vi "Save Data (SubVI).vi"(0 "Save Enable":bool, 5 "Save Interval [sec]":dbl=1.0 min=0.0 step=0.1, 7 "File Name":string, 9 "Folder Location":path, 11 "Data Array (Row)":string[](array[string]), 12 "Column Header Array":string[](array[string]), 13 "Title Block":string[][](array[string]), 14 "External Save Signal":bool) -> (4 "File Path":path, 8 "Row Count":u16, 15 "Save Error":errorcluster)   [LabVIEW 2012]
panel:
  # "SAVE DATA\nCreated by Blake Otting \nLast Update 7-11-2013"
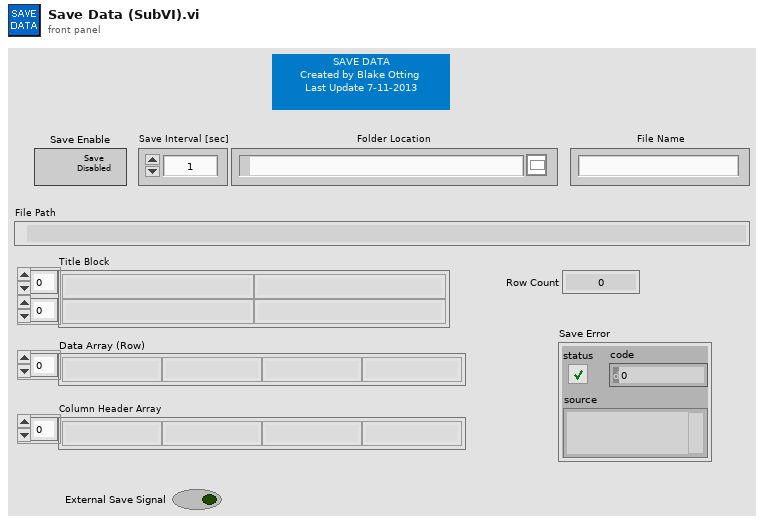
[diagram p1: front panel]
types:
  T1 = enum16{"open", "replace", "create", "open or create", "replace or create", "replace or create with confirmation"}
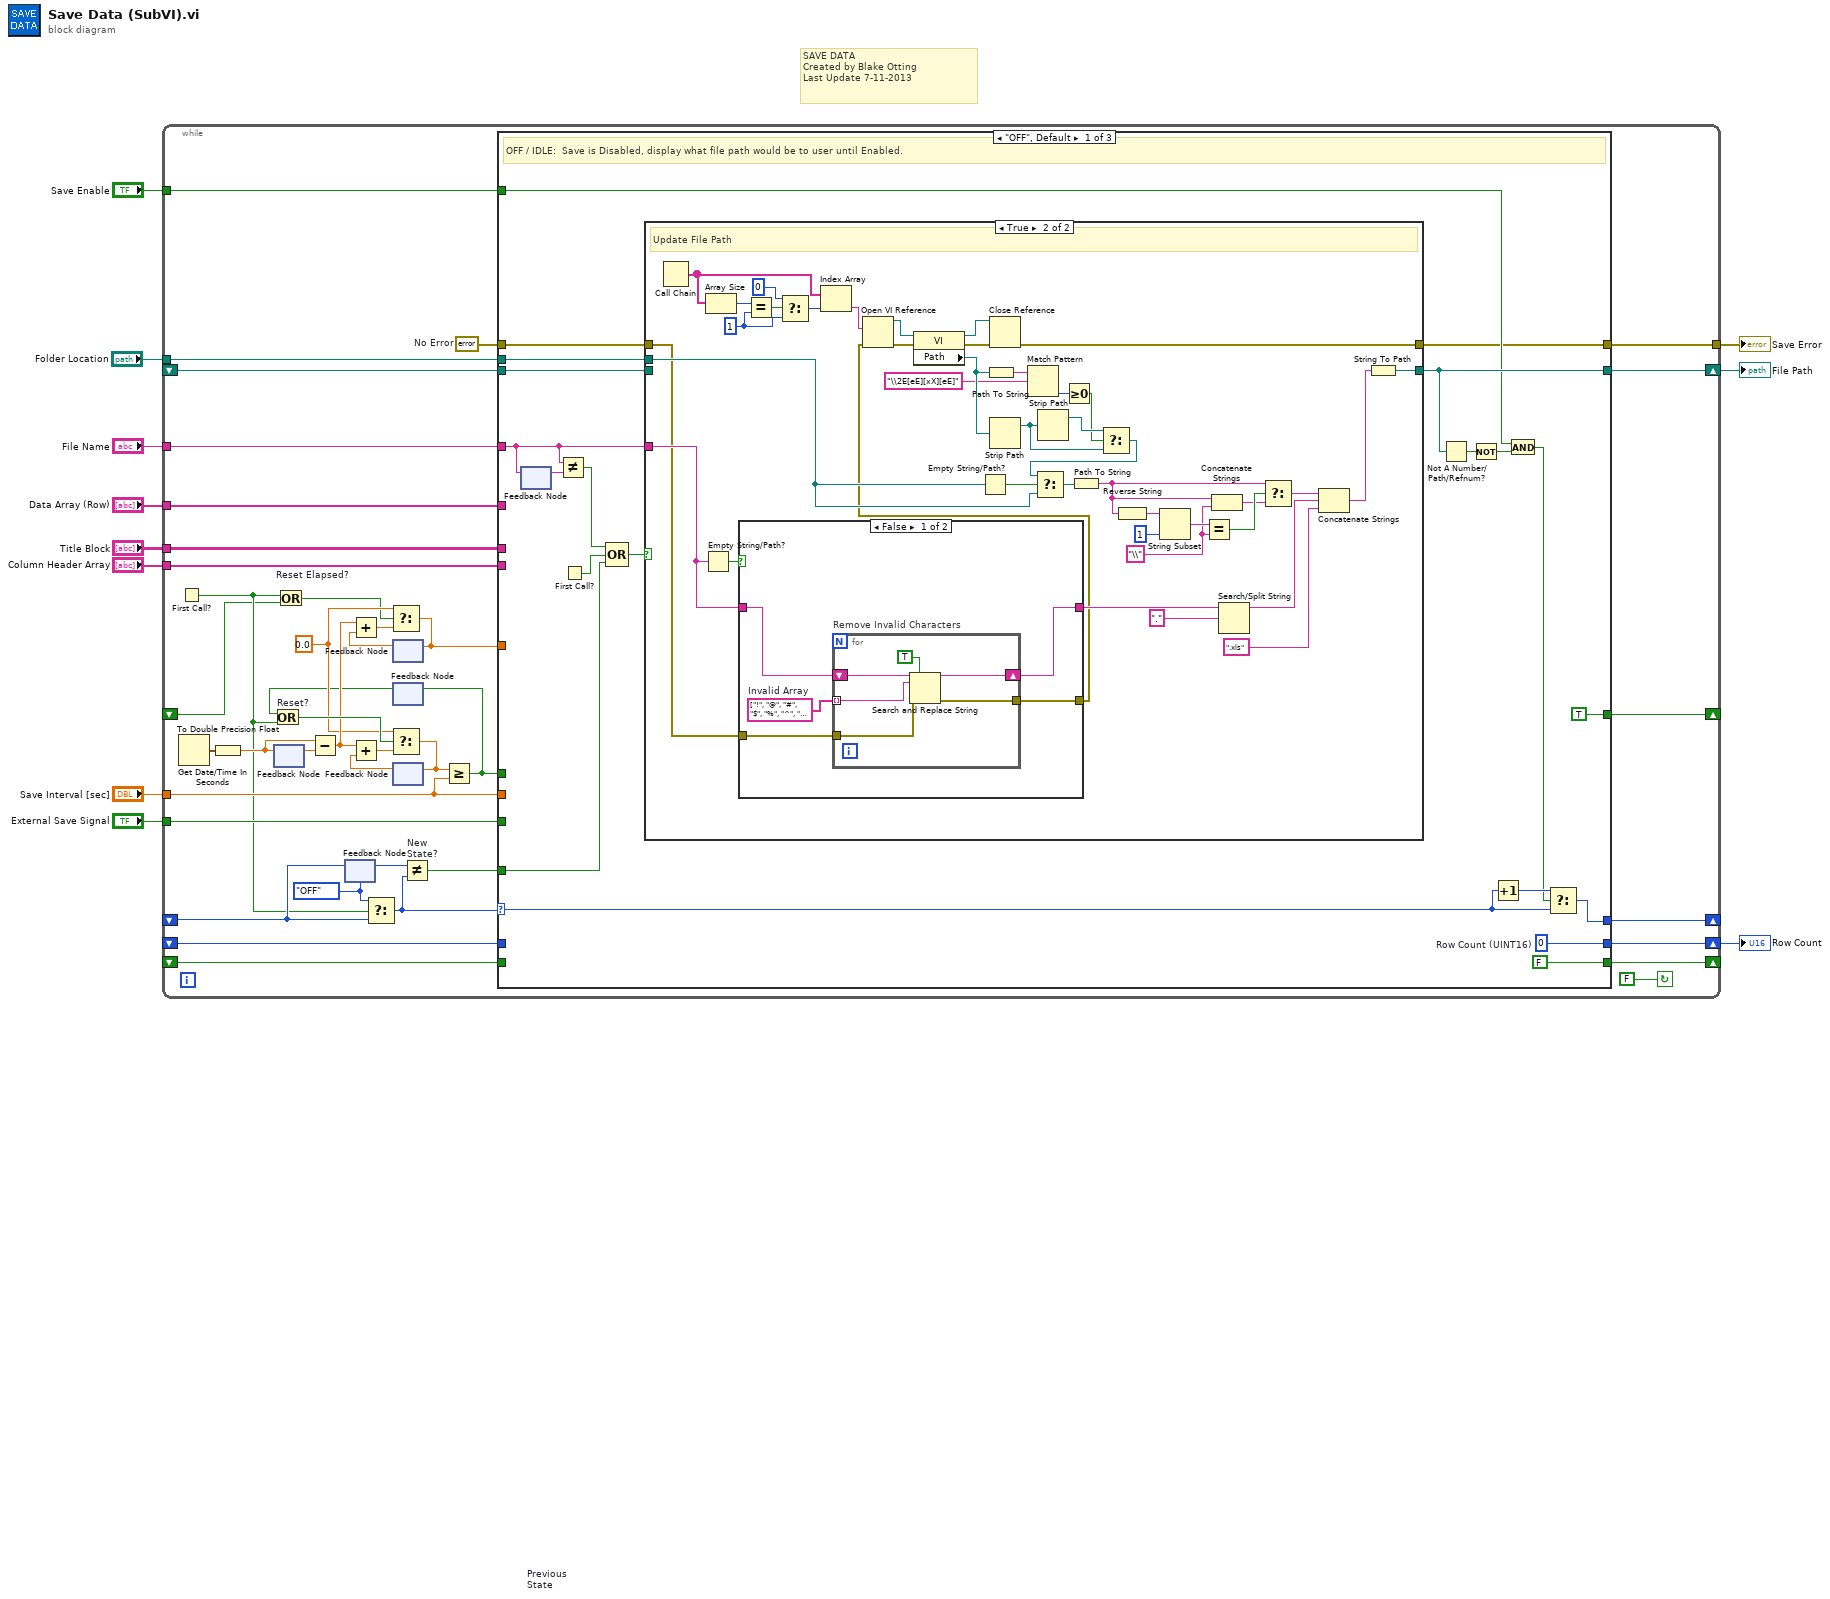
[diagram p0: block diagram]
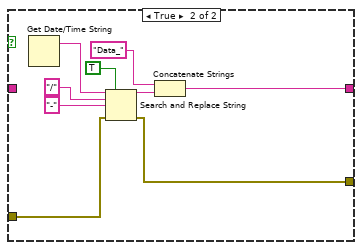
[diagram p3: hidden frame]
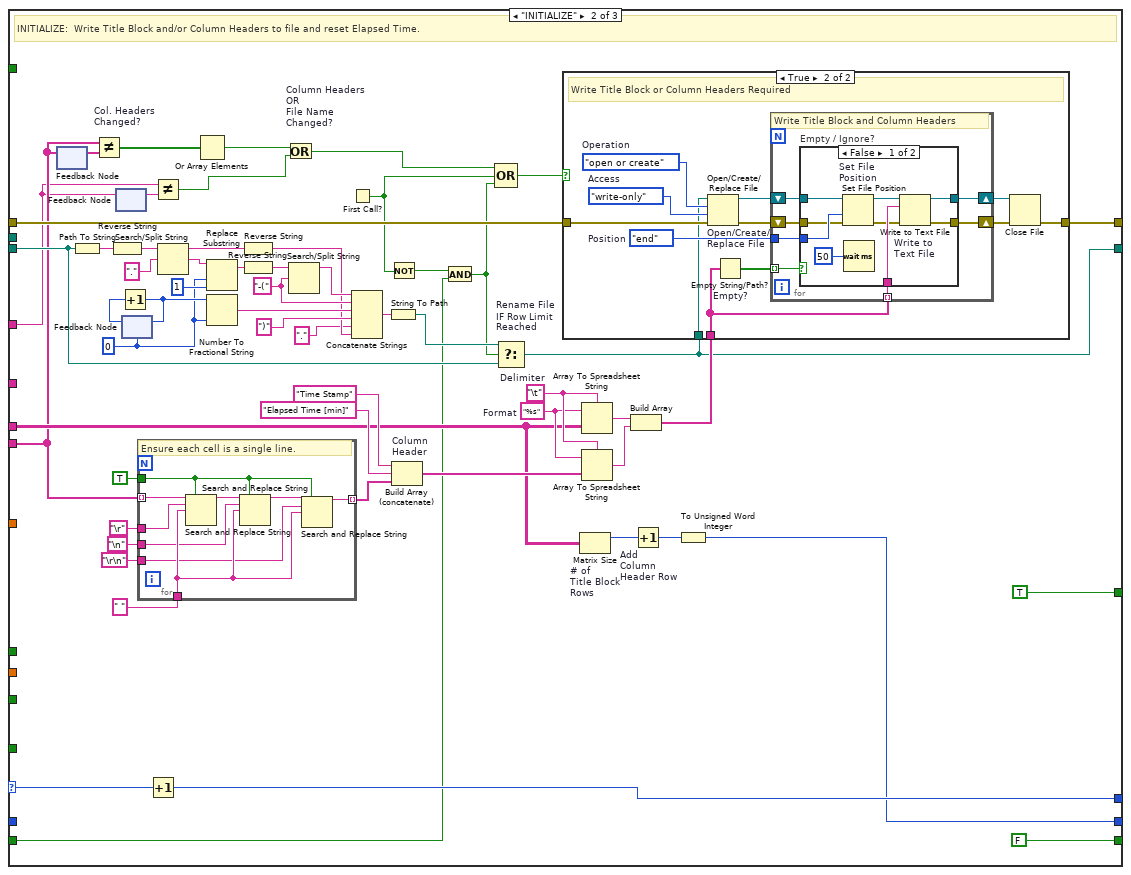
[diagram p4: hidden frame]
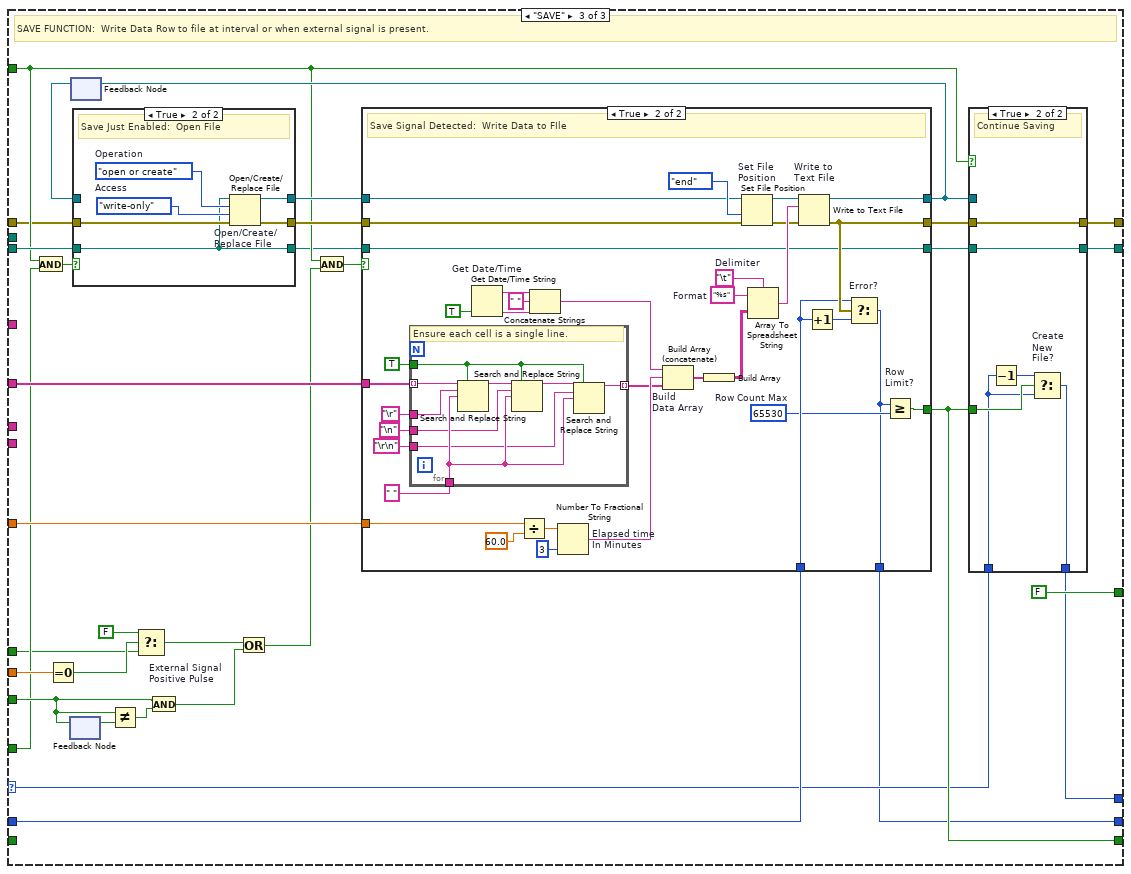
[diagram p7: hidden frame]
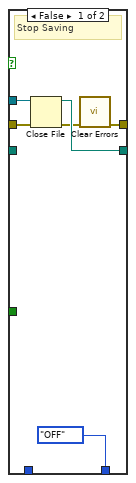
[diagram p9: hidden frame]
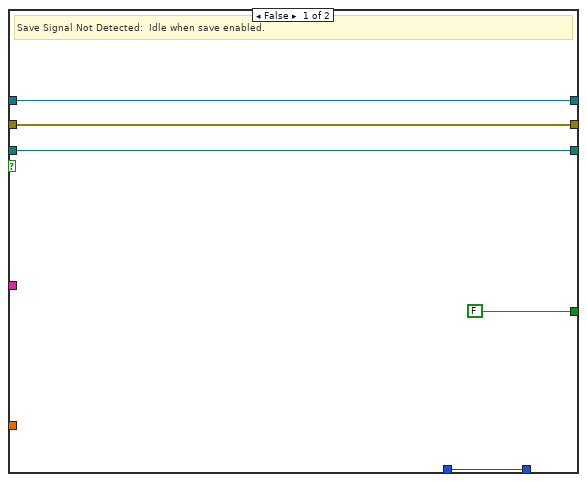
[diagram p10: hidden frame]
diagram:
  # "SAVE DATA\nCreated by Blake Otting \nLast Update 7-11-2013"
  n1 = while {
    tunnel: "Save Enable" -> [w25]
    shift-right: [w51] -> _
    shift-left: _ -> [w27]
    shift-right: [w50] -> w2
    shift-left: _ -> [w49]
    tunnel: "Title Block" -> [w48]
    tunnel: "Column Header Array" -> [w47]
    tunnel: "Data Array (Row)" -> [w46]
    shift-right: [w45] -> w3
    shift-left: _ -> [w44]
    shift-right: [w43] -> _
    shift-left: _ -> [w42]
    shift-right: [w30] -> _
    shift-left: _ -> [w15]
    tunnel: "Save Interval [sec]" -> [w19]
    tunnel: "Folder Location" -> [w29]
    tunnel: "File Name" -> [w12]
    tunnel: "External Save Signal" -> [w24]
    tunnel: [w28] -> w1
    stop <- FALSE continue-if-true
    w13 = errorcluster {"status"=FALSE, "code"=0, "source"=""}  # No Error
    w31 = 0.0 ("t")
    w26 = enum16{"OFF", "INITIALIZE", "SAVE"}."OFF"
    n2 = First Call?() -> (First Call?: T/F=w16:bool)
    n3 = Get Date/Time In Seconds() -> (seconds since 1Jan1904=w39:timestamp)
    n4 = To Double Precision Float(number=w39) -> (double precision float=w35:dbl)
    n5 = feedback #1() -> (w40:dbl)  [unwired: 1 in]
    n6 = feedback-in #1(w35) -> ()
    n7 = Or "Reset Elapsed?"(x=w16, y=w15) -> (x .or. y?=w14:bool)
    n8 = Subtract(x=w35, y=w40) -> (x-y=w32:dbl)
    n9 = feedback-in #2(w27) -> ()
    n10 = feedback #2 "Previous\nState"(w26) -> (w23:enum16{"OFF", "INITIALIZE", "SAVE"})
    n11 = Select(t=w26, s=w16, f=w27) -> (s? t:f=w22:enum16{"OFF", "INITIALIZE", "SAVE"})
    n12 = feedback #3() -> (w33:dbl)  [unwired: 1 in]
    n13 = Add(x=w32, y=w33) -> (x+y=w36:dbl)
    n14 = Select(t=w31, s=w14, f=w36) -> (s? t:f=w41:dbl)
    n15 = feedback-in #3(w41) -> ()
    n16 = feedback #4() -> (w17:bool)  [unwired: 1 in]
    n17 = Or "Reset?"(x=w17, y=w16) -> (x .or. y?=w37:bool)
    n18 = feedback #5() -> (w34:dbl)  [unwired: 1 in]
    n19 = Add(x=w32, y=w34) -> (x+y=w38:dbl)
    n20 = Select(t=w31, s=w37, f=w38) -> (s? t:f=w20:dbl)
    n21 = feedback-in #5(w20) -> ()
    n22 = Not Equal? "New\nState?"(x=w23, y=w22) -> (x != y?=w21:bool)
    n23 = Greater Or Equal?(x=w20, y=w19) -> (x >= y?=w18:bool)
    n24 = feedback-in #4(w18) -> ()
    n25 = case shown="\"OFF\", Default" w22 {
      selector: w22 -> [w72 w194 w240]
      tunnel: [w71 w193 w239] -> w51
      tunnel: w25 -> [w63 _ w245]
      tunnel: [w70 w184 w238] -> w50
      tunnel: w49 -> [_ _ w256]
      tunnel: w48 -> [_ w159 _]
      tunnel: w44 -> [w59 w183 w260]
      tunnel: w47 -> [_ w148 _]
      tunnel: w46 -> [_ _ w266]
      tunnel: w41 -> [_ _ w267]
      tunnel: [w64 w150 w262] -> w45
      tunnel: [FALSE FALSE w241] -> w43
      tunnel: w42 -> [_ w140 _]
      tunnel: [TRUE TRUE FALSE] -> w30
      tunnel: w29 -> [w68 _ _]
      tunnel: w12 -> [w54 w138 _]
      tunnel: w19 -> [_ _ w248]
      tunnel: w24 -> [_ _ w247]
      tunnel: [w60 w158 w263] -> w28
      tunnel: w21 -> [w57 _ w246]
      tunnel: w18 -> [_ _ w242]
      tunnel: w13 -> [w61 w151 w237]
      frame "OFF", Default {
        w70 = u16 0  # Row Count (UINT16)
        # "OFF / IDLE:  Save is Disabled, display what file path would be to user until Enabled."
        n26 = feedback #6() -> (w55:string)  [unwired: 1 in]
        n27 = feedback-in #6(w54) -> ()
        n28 = Not Equal?(x=w54, y=w55) -> (x != y?=w53:bool)
        n29 = First Call?() -> (First Call?: T/F=w58:bool)
        n30 = Compound Arithmetic op=OR(w53, w58, w57) -> (w56:bool)
        n31 = case shown="True" w56 {
          tunnel: w68 -> [_ w102]
          tunnel: [w74 w101] -> w64
          tunnel: w54 -> [_ w80]
          tunnel: w61 -> [w75 w77]
          tunnel: [w75 w78] -> w60
          tunnel: w59 -> [w74 _]
          frame False {
            # "File Path hasn't changed, do nothing."
          }
          frame True {
            w88 = 1 ("index")
            w108 = "\\"
            # "Update File Path"
            n32 = Call Chain() -> (call chain=w84:string[])
            n33 = Empty String/Path?(string/path=w80) -> (empty?=w100:bool)
            n34 = Array Size(array=w84) -> (size(s)=w87:i32)
            n35 = case shown="False" w100 {
              tunnel: w80 -> [w118 _]
              tunnel: [w117 w130] -> w99
              tunnel: w77 -> [w120 w129]
              tunnel: [w119 w128] -> w76
              frame False {
                w121 = string[] ["!", "@", "#", "$", "%", "^", "&", "*", "(", ")", "{", "}", "<", ">", "?", ":", ";", "\"", "'", "+"]  # Invalid Array
                n36 = for "Remove Invalid Characters" {
                  tunnel: w121 -> [w125] mode=indexing
                  shift-right: [w124] -> w117
                  shift-left: w118 -> [w126]
                  tunnel: w120 -> [w123]
                  tunnel: [w122] -> w119
                  n37 = Search and Replace String(replace all?=TRUE, input string=w126, search string=w125, error in=w123) -> (result string=w124:string, error out=w122:errorcluster)  [unwired: 4 in, 2 out]
                }
              }
              frame True {
                n38 = Get Date/Time String() -> (date string=w134:string)  [unwired: 3 in, 1 out]
                n39 = Search and Replace String(replace all?=TRUE, input string=w134, search string="/", replace string="-", error in=w129) -> (result string=w131:string, error out=w128:errorcluster)  [unwired: 3 in, 2 out]
                n40 = Concatenate Strings("Data_" ("search string/char (-)"), w131) -> (w130:string)
              }
            }
            n41 = Equal?(x=w87, y=w88) -> (x = y?=w85:bool)
            n42 = Select(t=0, s=w85, f=w88) -> (s? t:f=w86:i32)
            n43 = Index Array(array=w84, index=w86) -> (element=w92:string)
            n44 = Open VI Reference(vi path=w92, error in (no error)=w76) -> (vi reference=w91:refnum<vi>, error out=w90:errorcluster)  [unwired: 4 in]
            n45 = property class="VI"(reference=w91, error in=w90) -> (reference out=w94:refnum<vi>, error out=w93:errorcluster, "Path"=w96:path)
            n46 = Empty String/Path?(string/path=w102) -> (empty?=w105:bool)
            n47 = Path To String(path=w96) -> (string=w82:string)
            n48 = Close Reference(reference=w94, error in (no error)=w93) -> (error out=w78:errorcluster)
            n49 = Strip Path(path=w96) -> (stripped path=w97:path)  [unwired: 1 out]
            n50 = Match Pattern(string=w82, regular expression="\\2E[eE][xX][eE]") -> (offset past match=w81:i32)  [unwired: 1 in, 3 out]
            n51 = Strip Path(path=w97) -> (stripped path=w98:path)  [unwired: 1 out]
            n52 = Greater Or Equal To 0?(x=w81) -> (x >= 0?=w95:bool)
            n53 = Select(t=w98, s=w95, f=w97) -> (s? t:f=w79:path)
            n54 = Select(t=w79, s=w105, f=w102) -> (s? t:f=w104:path)
            n55 = Path To String(path=w104) -> (string=w103:string)
            n56 = Reverse String(1:w103) -> (0:w112:string)
            n57 = String Subset(string=w112, length (rest)=1) -> (substring=w110:string)  [unwired: 1 in]
            n58 = Equal?(x=w110, y=w108) -> (x = y?=w109:bool)
            n59 = Concatenate Strings(w103, w108) -> (w107:string)
            n60 = Search/Split String(string=w99, search string/char (-)=".") -> (substring before match=w113:string)  [unwired: 1 in, 2 out]
            n61 = Select(t=w103, s=w109, f=w107) -> (s? t:f=w106:string)
            n62 = Concatenate Strings(w106, w113, ".xls" ("string")) -> (w115:string)
            n63 = String To Path(string=w115) -> (path=w101:path)
          }
        }
        n64 = Not A Number/Path/Refnum?(number/path/refnum=w64) -> (NaN/Path/Refnum?=w65:bool)
        n65 = Not(x=w65) -> (.not. x?=w66:bool)
        n66 = Increment(x=w72) -> (x+1=w73:enum16{"OFF", "INITIALIZE", "SAVE"})
        n67 = And(x=w63, y=w66) -> (x .and. y?=w62:bool)
        n68 = Select(t=w73, s=w62, f=w72) -> (s? t:f=w71:enum16{"OFF", "INITIALIZE", "SAVE"})
      }
      frame "INITIALIZE" {
        w164 = u8 0
        w172 = "-("
        w192 = "\t"  # Delimiter
        w191 = "%s"  # Format
        # "INITIALIZE:  Write Title Block and/or Column Headers to file and reset Elapsed Time."
        n69 = feedback #7() -> (w149:string[])  [unwired: 1 in]
        n70 = feedback-in #7(w148) -> ()
        n71 = Path To String(path=w183) -> (string=w175:string)
        n72 = Not Equal? "Col. Headers\nChanged?"(x=w148, y=w149) -> (x != y?=w147:bool[])
        n73 = Reverse String(1:w175) -> (0:w176:string)
        n74 = feedback #8() -> (w139:string)  [unwired: 1 in]
        n75 = feedback-in #8(w138) -> ()
        n76 = feedback #9(w164) -> (w170:u8)
        n77 = Increment(x=w170) -> (x+1=w171:u8)
        n78 = feedback-in #9(w171) -> ()
        n79 = for {
          tunnel: w148 -> [w234] mode=indexing
          tunnel: TRUE -> [w232]
          tunnel: [w230] -> w152 mode=indexing
          tunnel: " " ("replace string (\"\")") -> [w229]
          tunnel: "\r" -> [w228]
          tunnel: "\n" -> [w227]
          tunnel: "\r\n" -> [w226]
          # "Ensure each cell is a single line."
          n80 = Search and Replace String(replace all?=w232, input string=w234, search string=w228, replace string=w229) -> (result string=w233:string)  [unwired: 4 in, 3 out]
          n81 = Search and Replace String(replace all?=w232, input string=w233, search string=w227, replace string=w229) -> (result string=w231:string)  [unwired: 4 in, 3 out]
          n82 = Search and Replace String(replace all?=w232, input string=w231, search string=w226, replace string=w229) -> (result string=w230:string)  [unwired: 4 in, 3 out]
        }
        n83 = Increment(x=w194) -> (x+1=w193:enum16{"OFF", "INITIALIZE", "SAVE"})
        n84 = Not Equal?(x=w138, y=w139) -> (x != y?=w137:bool)
        n85 = Search/Split String(string=w176, search string/char (-)=".") -> (substring before match=w177:string, match + rest of string=w178:string)  [unwired: 2 out]
        n86 = Or Array Elements(Boolean array=w147) -> (logical OR=w146:bool)
        n87 = Replace Substring(2:1 ("length (len. of substring)"), 3:w164, 5:w178) -> (1:w179:string)  [unwired: 2 out]
        n88 = Number To Fractional String(number=w171, precision (6)=w164) -> (F-format string=w181:string)  [unwired: 2 in]
        n89 = Reverse String(1:w177) -> (0:w167:string)
        n90 = Reverse String(1:w179) -> (0:w173:string)
        n91 = Or "Column Headers\nOR\nFile Name\nChanged?"(x=w146, y=w137) -> (x .or. y?=w145:bool)
        n92 = Search/Split String(string=w173, search string/char (-)=w172) -> (substring before match=w169:string)  [unwired: 1 in, 2 out]
        n93 = First Call?() -> (First Call?: T/F=w144:bool)
        n94 = Concatenate Strings(w169, w172, w181, ")", "." ("search string/char (-)"), w167) -> (w166:string)
        n95 = String To Path(string=w166) -> (path=w182:path)
        n96 = Not(x=w144) -> (.not. x?=w141:bool)
        n97 = Build Array (concatenate) "Column\nHeader"("Time Stamp", "Elapsed Time [min]", w152) -> (w189:string[])
        n98 = And(x=w141, y=w140) -> (x .and. y?=w143:bool)
        n99 = Compound Arithmetic op=OR(w145, w144, w143) -> (w142:bool)
        n100 = Select "Rename File\nIF Row Limit\nReached"(t=w182, s=w143, f=w183) -> (s? t:f=w150:path)
        n101 = Matrix Size "# of\nTitle Block\nRows"(0:w159) -> (1:w186:i32)  [unwired: 1 out]
        n102 = Array To Spreadsheet String(delimiter (Tab)=w192, array=w159, 3:w191) -> (spreadsheet string=w188:string)
        n103 = Array To Spreadsheet String(delimiter (Tab)=w192, array=w189, 3:w191) -> (spreadsheet string=w187:string)
        n104 = Build Array(w188, w187) -> (w161:string[])
        n105 = case shown="True" w142 {
          tunnel: w161 -> [_ w202]
          tunnel: [w195 w198] -> w158
          tunnel: w151 -> [w195 w197]
          tunnel: w150 -> [_ w196]
          frame False {
            # "No need to write Title Block or Column Headers"
          }
          frame True {
            w205 = enum16{"read/write", "read-only", "write-only"}."write-only"  # Access
            w207 = enum16{"start", "end", "current"}."end"  # Position
            w206 = T1."open or create"  # Operation
            # "Write Title Block or Column Headers Required"
            n106 = Open/Create/Replace File "Open/Create/\nReplace File"(file path (use dialog)=w196, error in=w197, operation (0:open)=w206, access (0:read/write)=w205) -> (refnum out=w204:refnum<file>, error out=w203:errorcluster)  [unwired: 2 in, 1 out]
            n107 = Empty String/Path? "Empty?"(string/path=w202) -> (empty?=w201:bool[])
            n108 = for {
              tunnel: w202 -> [w213] mode=indexing
              tunnel: w207 -> [w212]
              shift-right: [w214] -> w199
              shift-left: w203 -> [w211]
              shift-right: [w209] -> w200
              shift-left: w204 -> [w210]
              tunnel: w201 -> [w208] mode=indexing
              # "Write Title Block and Column Headers"
              n109 = case "Empty / Ignore?" shown="False" w208 {
                tunnel: [w222 w225] -> w214
                tunnel: [w221 w224] -> w209
                tunnel: w213 -> [w220 _]
                tunnel: w212 -> [w219 _]
                tunnel: w211 -> [w218 w225]
                tunnel: w210 -> [w217 w224]
                frame False {
                  n110 = Set File Position "Set File \nPosition"(refnum=w217, from (0:start)=w219, error in=w218) -> (refnum out=w215:refnum<file>, error out=w216:errorcluster)  [unwired: 1 in]
                  n111 = Wait (ms)(milliseconds to wait=u32 50) -> ()  [unwired: 1 out]
                  n112 = Write to Text File "Write to \nText File"(file (use dialog)=w215, text=w220, error in=w216) -> (refnum out=w221:refnum<file>, error out=w222:errorcluster)  [unwired: 1 in, 1 out]
                }
                frame True {
                }
              }
            }
            n113 = Close File(refnum=w200, error in=w199) -> (error out=w198:errorcluster)  [unwired: 1 out]
          }
        }
        n114 = Increment "Add\nColumn\nHeader Row"(x=w186) -> (x+1=w185:i32)
        n115 = To Unsigned Word Integer(number=w185) -> (unsigned 16bit integer=w184:u16)
      }
      frame "SAVE" {
        # "SAVE FUNCTION:  Write Data Row to file at interval or when external signal is present."
        n116 = And(x=w245, y=w246) -> (x .and. y?=w249:bool)
        n117 = Equal To 0?(x=w248) -> (x = 0?=w253:bool)
        n118 = feedback-in #10(w247) -> ()
        n119 = feedback #10() -> (w252:bool)  [unwired: 1 in]
        n120 = feedback #11() -> (w258:refnum<file>)  [unwired: 1 in]
        n121 = case shown="True" w249 {
          tunnel: w260 -> [w268 w271]
          tunnel: [w269 w274] -> w259
          tunnel: w258 -> [w270 _]
          tunnel: [w270 w273] -> w257
          tunnel: w237 -> [w269 w272]
          tunnel: [w268 w271] -> w235
          frame False {
            # "File Previously Opened:  Use Ref"
          }
          frame True {
            w275 = enum16{"read/write", "read-only", "write-only"}."write-only"  # Access
            w276 = T1."open or create"  # Operation
            # "Save Just Enabled:  Open File"
            n122 = Open/Create/Replace File "Open/Create/\nReplace File"(file path (use dialog)=w271, error in=w272, operation (0:open)=w276, access (0:read/write)=w275) -> (refnum out=w273:refnum<file>, error out=w274:errorcluster)  [unwired: 2 in, 1 out]
          }
        }
        n123 = Not Equal?(x=w247, y=w252) -> (x != y?=w251:bool)
        n124 = Select(t=FALSE, s=w253, f=w242) -> (s? t:f=w254:bool)
        n125 = And "External Signal\nPositive Pulse"(x=w247, y=w251) -> (x .and. y?=w250:bool)
        n126 = Or(x=w254, y=w250) -> (x .or. y?=w244:bool)
        n127 = And(x=w245, y=w244) -> (x .and. y?=w243:bool)
        n128 = case shown="True" w243 {
          tunnel: w267 -> [_ w309]
          tunnel: w266 -> [_ w302]
          tunnel: w259 -> [w293 w315]
          tunnel: [w293 w300] -> w264
          tunnel: w257 -> [w292 w314]
          tunnel: [w292 w311] -> w261
          tunnel: w256 -> [w291 w298]
          tunnel: [w291 w296] -> w238
          tunnel: [FALSE w295] -> w241
          tunnel: [w289 w294] -> w236
          tunnel: w235 -> [w289 w294]
          frame False {
            # "Save Signal Not Detected:  Idle when save enabled."
          }
          frame True {
            w297 = u16 65530  # Row Count Max
            w317 = "\t"  # Delimiter
            w320 = "%s"  # Format
            # "Save Signal Detected:  Write Data to FIle"
            n129 = for {
              tunnel: w302 -> [w337] mode=indexing
              tunnel: TRUE -> [w335]
              tunnel: [w333] -> w301 mode=indexing
              tunnel: " " ("replace string (\"\")") -> [w332]
              tunnel: "\r" -> [w331]
              tunnel: "\n" -> [w330]
              tunnel: "\r\n" -> [w329]
              # "Ensure each cell is a single line."
              n130 = Search and Replace String(replace all?=w335, input string=w337, search string=w331, replace string=w332) -> (result string=w336:string)  [unwired: 4 in, 3 out]
              n131 = Search and Replace String(replace all?=w335, input string=w336, search string=w330, replace string=w332) -> (result string=w334:string)  [unwired: 4 in, 3 out]
              n132 = Search and Replace String(replace all?=w335, input string=w334, search string=w329, replace string=w332) -> (result string=w333:string)  [unwired: 4 in, 3 out]
            }
            n133 = Get Date/Time String "Get Date/Time"(want seconds? (F)=TRUE) -> (date string=w321:string, time string=w324:string)  [unwired: 2 out]
            n134 = Divide(x=w309, y=60.0) -> (x/y=w308:dbl)
            n135 = Concatenate Strings(w321, " " ("string"), w324) -> (w325:string)
            n136 = Number To Fractional String "Elapsed time\nIn Minutes"(number=w308, precision (6)=i16 3) -> (F-format string=w318:string)  [unwired: 2 in]
            n137 = Build Array (concatenate) "Build\nData Array"(w325, w318, w301) -> (w326:string[])
            n138 = Build Array(w326) -> (w327:string[][])
            n139 = Set File Position "Set File \nPosition"(refnum=w314, from (0:start)=enum16{"start", "end", "current"}."end", error in=w315) -> (refnum out=w312:refnum<file>, error out=w313:errorcluster)  [unwired: 1 in]
            n140 = Array To Spreadsheet String(delimiter (Tab)=w317, array=w327, 3:w320) -> (spreadsheet string=w316:string)
            n141 = Write to Text File "Write to \nText File"(file (use dialog)=w312, text=w316, error in=w313) -> (refnum out=w311:refnum<file>, error out=w300:errorcluster)  [unwired: 1 in, 1 out]
            n142 = Increment(x=w298) -> (x+1=w299:u16)
            n143 = Select "Error?"(t=w298, s=w300, f=w299) -> (s? t:f=w296:u16)
            n144 = Greater Or Equal? "Row\nLimit?"(x=w296, y=w297) -> (x >= y?=w295:bool)
          }
        }
        n145 = feedback-in #11(w261) -> ()
        n146 = case shown="True" w245 {
          tunnel: w261 -> [w280 _]
          tunnel: w264 -> [w282 w288]
          tunnel: [w277 w288] -> w263
          tunnel: [w281 w283] -> w262
          tunnel: w241 -> [_ w286]
          tunnel: w240 -> [_ w285]
          tunnel: [enum16{"OFF", "INITIALIZE", "SAVE"}."OFF" w284] -> w239
          tunnel: w236 -> [_ w283]
          frame False {
            # "Stop Saving"
            n147 = Close File(refnum=w280, error in=w282) -> (path=w281:path, error out=w278:errorcluster)
            n148 = call <vilib>:"Clear Errors.vi"("error in (no error)"=w278) -> ("error out"=w277:errorcluster)  [unwired: 6 in]
          }
          frame True {
            # "Continue Saving"
            n149 = Decrement(x=w285) -> (x-1=w287:enum16{"OFF", "INITIALIZE", "SAVE"})
            n150 = Select "Create\nNew\nFile?"(t=w287, s=w286, f=w285) -> (s? t:f=w284:enum16{"OFF", "INITIALIZE", "SAVE"})
          }
        }
      }
    }
  }
  "File Path" <- w3
  "Row Count" <- w2
  "Save Error" <- w1
